vi "Tree_Rename.vi"(9 "Tree in":string, 10 "Panel":refnum<vi>, 11 "TreeControl in":refnum<vi>) -> ()   [LabVIEW 2020]
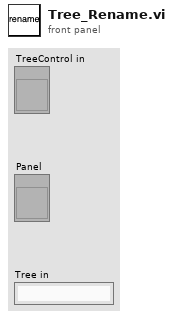
[diagram p1: front panel]
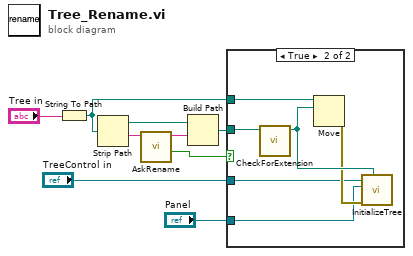
[diagram p0: block diagram]
diagram:
  n1 = String To Path(string="Tree in") -> (path=w2:path)
  n2 = Strip Path(path=w2) -> (stripped path=w3:path, name=w6:string)
  n3 = call "AskRename.vi"("name"=w6) -> ("OK?"=w5:bool, "name 2"=w7:string)  [unwired: 9 in]
  n4 = Build Path(base path=w3, name or relative path=w7) -> (appended path=w4:path)
  n5 = case shown="True" w5 {
    tunnel: w2 -> [_ w15]
    tunnel: w4 -> [_ w14]
    tunnel: "Panel" -> [_ w11]
    tunnel: "TreeControl in" -> [_ w10]
    frame False {
    }
    frame True {
      n6 = call "CheckForExtension.vi"("selected path"=w14) -> ("dup file"=w13:path)  [unwired: 10 in]
      n7 = Move(source path=w15, 10:w13) -> (error out=w12:errorcluster)  [unwired: 3 in, 2 out]
      n8 = call "InitializeTree.vi"("Selected File"=w13, "error in (no error)"=w12, "Panel"=w11, "TreeControl in"=w10) -> ()  [unwired: 7 in, 1 out]
    }
  }
